vi "Configure Source (Level).vi"(0 "VISA resource name":refnum<visa-resource-name>, 1 "Current Level (0 A)":dbl, 5 "Source Measure Unit Channel (0: Channel A)":i32(ring) items=["Channel A", "Channel B"], 7 "Level Type (1: Voltage)":i32(ring)=1 items=["Current", "Voltage"], 11 "error in (no error)":errorcluster, 12 "Voltage Level (0 V)":dbl) -> (4 "VISA resource name out":refnum<visa-resource-name>, 15 "error out":errorcluster)   [LabVIEW 2015, in "Keithley 2600 Series.lvlib"]
doc: "Configures the source level."
uses:
  Keithley 2600 Series.lvlib
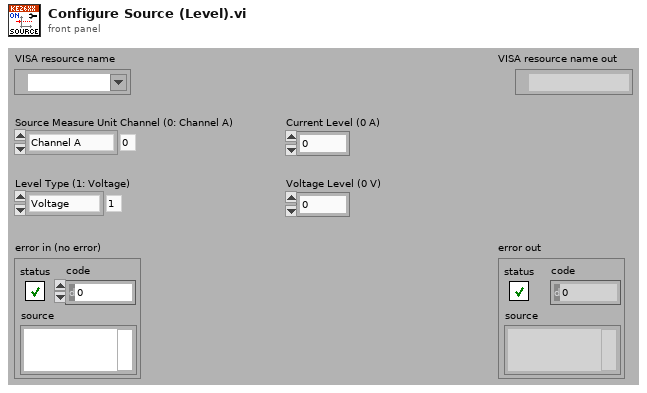
[diagram p1: front panel]
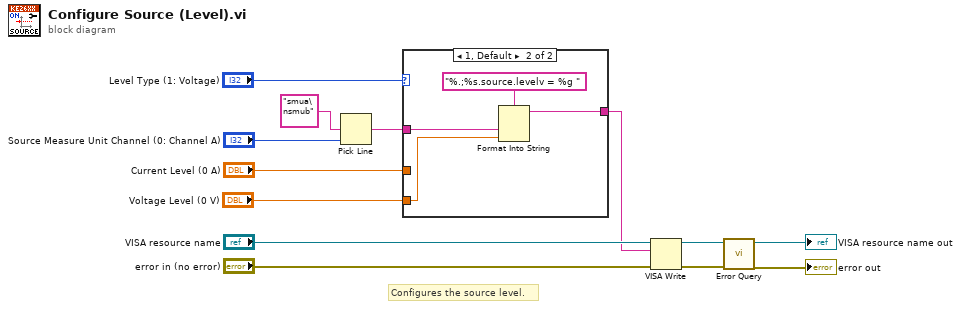
[diagram p0: block diagram]
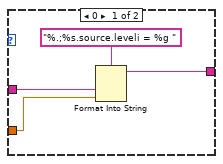
[diagram p2: hidden frame]
diagram:
  # "Configures the source level."
  n1 = Pick Line(multi-line string="smua\nsmub", line index="Source Measure Unit Channel (0: Channel A)") -> (output string=w5:string)  [unwired: 1 in]
  n2 = case shown="1, Default" "Level Type (1: Voltage)" {
    tunnel: w5 -> [w16 w20]
    tunnel: "Current Level (0 A)" -> [w14 _]
    tunnel: "Voltage Level (0 V)" -> [_ w18]
    tunnel: [w15 w19] -> w1
    frame 0 {
      n3 = Format Into String(format string="%.;%s.source.leveli = %g ", w16, w14) -> (resulting string=w15:string)  [unwired: 2 in, 1 out]
    }
    frame 1, Default {
      n4 = Format Into String(format string="%.;%s.source.levelv = %g ", w20, w18) -> (resulting string=w19:string)  [unwired: 2 in, 1 out]
    }
  }
  n5 = VISA Write(VISA resource name="VISA resource name", write buffer=w1, error in (no error)="error in (no error)") -> (VISA resource name out=w11:refnum<visa-resource-name>, error out=w10:errorcluster)  [unwired: 1 out]
  n6 = call "Error Query.vi"("error in (no error)"=w10, "VISA resource name"=w11) -> ("error out"=→"error out":errorcluster, "VISA resource name out"=→"VISA resource name out":refnum<visa-resource-name>)  [unwired: 6 in, 2 out]
